vi "Configure DAQ Trigger.vi"(8 "error in (no error)":errorcluster, 9 "FGEN Channels":string[](array[string]), 10 "FGEN Resource":refnum<k15>, 11 "DAQmx Tasks In":T1) -> (0 "error out":errorcluster, 3 "DAQmx Tasks Out":T1)   [LabVIEW 2025]
uses:
  <vilib>/DAQmx/configure/trigger.llb/DAQmx Start Trigger (Digital Edge).vi
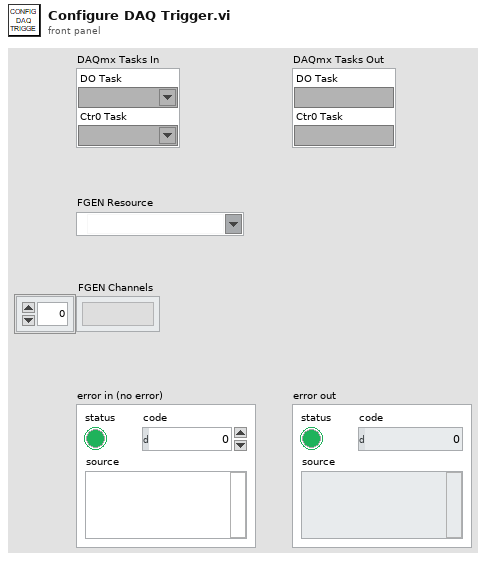
[diagram p1: front panel]
types:
  T1 = cluster{"DO Task":refnum<k21>, "Ctr0 Task":refnum<k21>}
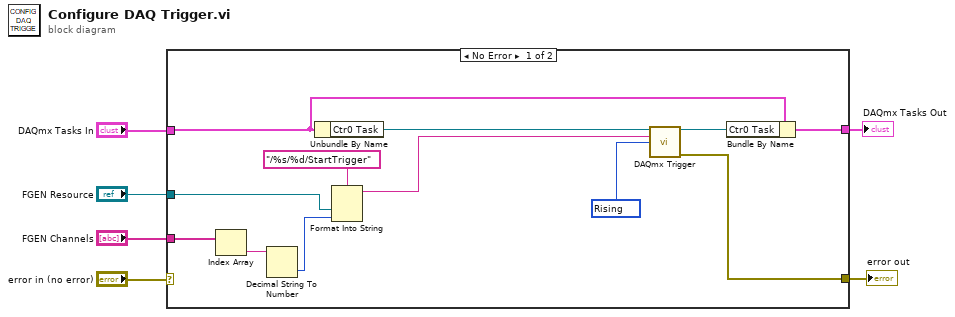
[diagram p0: block diagram]
diagram:
  n1 = case shown="No Error" "error in (no error)" {
    selector: "error in (no error)" -> [_ w19]
    tunnel: [w9 w19] -> w6
    tunnel: "DAQmx Tasks In" -> [w7 _]
    tunnel: [w8 _] -> w3
    tunnel: "FGEN Resource" -> [w15 _]
    tunnel: "FGEN Channels" -> [w16 _]
    frame No Error {
      w11 = 10280 items=["Rising"=10280, "Falling"=10171] ("edge")
      n2 = Index Array(array=w16) -> (element=w14:string)  [unwired: 1 in]
      n3 = Decimal String To Number(string=w14) -> (number=w13:i32)  [unwired: 2 in, 1 out]
      n4 = Unbundle By Name(w7) -> ("Ctr0 Task"=w10:refnum<k21>)
      n5 = Format Into String(format string="/%s/%d/StartTrigger", w15, w13) -> (resulting string=w12:string)  [unwired: 2 in, 1 out]
      n6 = call-poly <vilib>:"DAQmx Trigger.vi"("task/channels in"=w10, "source"=w12, "edge"=w11) -> ("task out"=w18:refnum<k21>, "error out"=w9:errorcluster)  [unwired: 11 in]
      n7 = Bundle By Name(cluster=w7, "Ctr0 Task"=w18) -> (w8:T1)
    }
    frame Error {
    }
  }
  "error out" <- w6
  "DAQmx Tasks Out" <- w3
